vi "Insert VIs by Pattern.vi"(7 "Application in":refnum<vi>, 8 "error in":errorcluster, 10 "VI Type":T1, 11 "Library In":refnum<class "Library.lvclass">) -> (0 "error out":errorcluster, 3 "Library Out":refnum<class "Library.lvclass">)   [LabVIEW 2020, in "Panther Dashboard.lvlib" / "Library.lvclass"]
uses:
  Library.lvclass
  LabVIEWItem/Item Type--enum.ctl
  Library.lvclass/Library.ctl
  Read Library Ref.vi
  LabVIEWItem/LabVIEWItem.lvclass
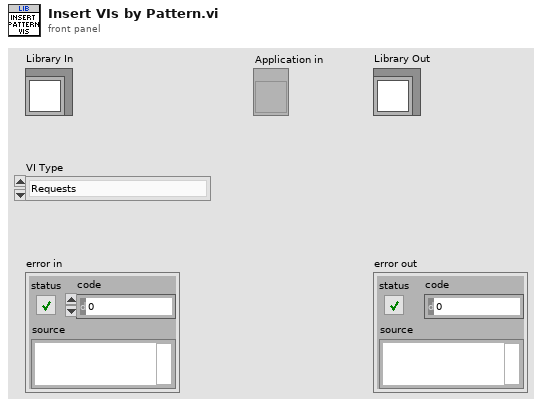
[diagram p1: front panel]
types:
  T1 = typedef "Panther Dashboard.lvlib/LabVIEWItem.lvclass/Item Type--enum.ctl" = enum16{"Requests", "Broadcasts", "Request and Wait for Reply", "Round Trip", "» Public API VIs", "» Constant VIs", "» Error VIs", "Module", "Project", "No Drag Selection"}
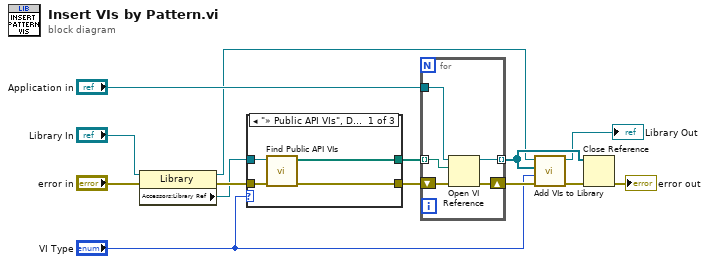
[diagram p0: block diagram]
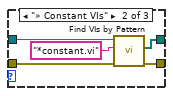
[diagram p2: hidden frame]
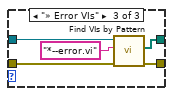
[diagram p3: hidden frame]
diagram:
  n1 = property class="Library"(reference="Library In", error in="error in") -> (reference out=w2:refnum<class "Library.lvclass">, error out=w13:errorcluster, "Accessors:Library Ref"=w7:refnum<vi>)
  n2 = case shown="\"» Public API VIs\", Default" "VI Type" {
    tunnel: w7 -> [w16 w20 w24]
    tunnel: [w15 w19 w26] -> w5
    tunnel: w13 -> [w18 w23 w28]
    tunnel: [w17 w22 w27] -> w11
    frame "» Public API VIs", Default {
      n3 = call "Find Public API VIs.vi"("error in"=w18, "Library in"=w16) -> ("error out"=w17:errorcluster, "Public API VIs Paths"=w15:path[])  [unwired: 8 in]
    }
    frame "» Constant VIs" {
      n4 = call "Find VIs by Pattern.vi"("error in"=w23, "pattern"="*constant.vi", "Library in"=w20) -> ("error out"=w22:errorcluster, "All Files in Dir"=w19:path[])  [unwired: 6 in, 1 out]
    }
    frame "» Error VIs" {
      n5 = call "Find VIs by Pattern.vi"("error in"=w28, "pattern"="*--error.vi", "Library in"=w24) -> ("error out"=w27:errorcluster, "All Files in Dir"=w26:path[])  [unwired: 6 in, 1 out]
    }
  }
  n6 = for {
    tunnel: "Application in" -> [w31]
    tunnel: w5 -> [w30] mode=indexing
    tunnel: [w29] -> w3 mode=indexing
    shift-right: [w32] -> w9
    shift-left: w11 -> [w33]
    n7 = Open VI Reference(application reference (local)=w31, vi path=w30, error in (no error)=w33) -> (vi reference=w29:refnum<vi>, error out=w32:errorcluster)  [unwired: 3 in]
  }
  n8 = call "Add VIs to Library.vi"("error in"=w9, "Event Type"="VI Type", "Event VIs"=w3, "Library In"=w2) -> ("error out"=w12:errorcluster, "Library Out"=→"Library Out":refnum<class "Library.lvclass">)  [unwired: 6 in]
  n9 = Close Reference(reference=w3, error in (no error)=w12) -> (error out=→"error out":errorcluster)
